vi "Write Status String.vi"(8 "error in (no error)":errorcluster, 10 "Status String":string, 11 "Update Status Display in":refnum<class "Update Status Display.lvclass">) -> (0 "error out":errorcluster, 3 "Update Status Display out":refnum<class "Update Status Display.lvclass">)   [LabVIEW 2016, in "Generic UI Actor.lvlib" / "Update Status Display.lvclass"]
uses:
  <userlib>/Common Components/User Interface/Messages/Update Status Display/Update Status Display.lvclass
  <userlib>/Common Components/User Interface/Messages/Update Status Display/Update Status Display.lvclass/Update Status Display.ctl
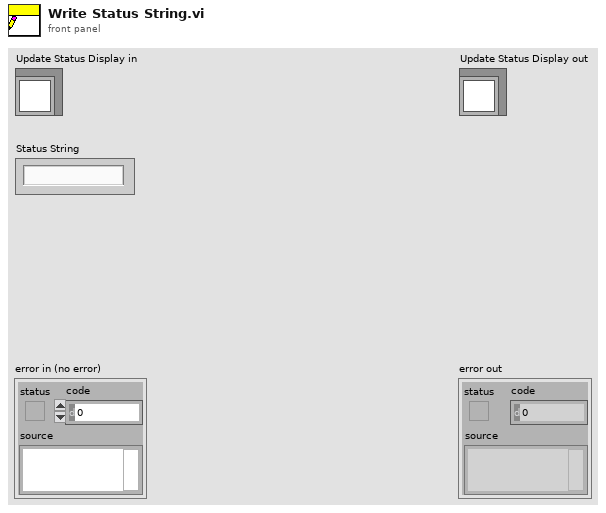
[diagram p1: front panel]
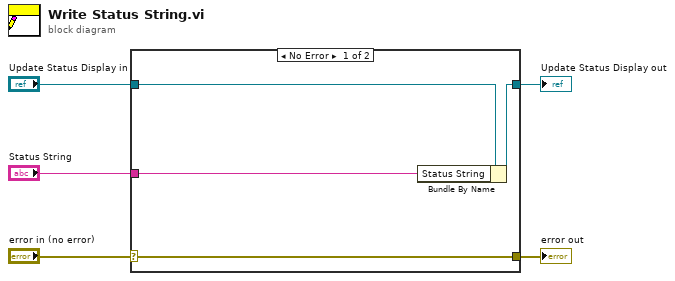
[diagram p0: block diagram]
diagram:
  n1 = case shown="No Error" "error in (no error)" {
    selector: "error in (no error)" -> [w9 w10]
    tunnel: [w9 w10] -> w4
    tunnel: [w7 w11] -> w2
    tunnel: "Update Status Display in" -> [w8 w11]
    tunnel: "Status String" -> [w6 _]
    frame No Error {
      n2 = Bundle By Name(cluster=w8, "Status String"=w6) -> (w7:refnum<class "Update Status Display.lvclass">)
    }
    frame Error {
    }
  }
  "error out" <- w4
  "Update Status Display out" <- w2
